vi "Sample_Data_Compute.vi"(8 "Data Array 2":dbl[][](array[numeric]), 11 "Data Array 1":dbl[][](array[numeric])) -> (0 "Cam2_Stats":cluster{"Mean_Area":i32, "Img_Count":u32} caption="Camera 2", 1 "Cam1_Stats":cluster{"Mean_Area":i32, "Img_Count":u32} caption="Camera 1", 3 "summaryData":T1)   [LabVIEW 2022 SP3]
uses:
  <vilib>/Analysis/NI_AALBase.lvlib
panel:
  in  "summaryData":T1
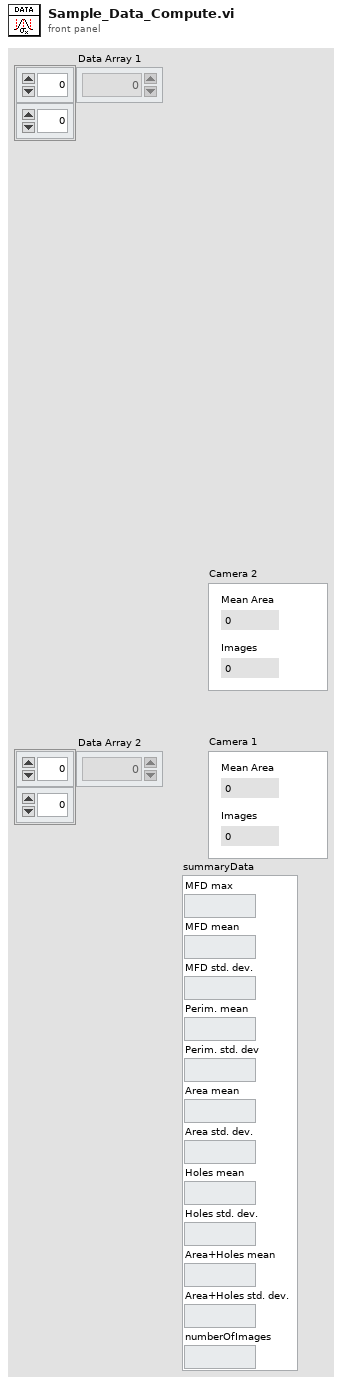
[diagram p1: front panel]
types:
  T1 = cluster{"MFD max":string, "MFD mean":string, "MFD std. dev.":string, "Perim. mean":string, "Perim. std. dev":string, "Area mean":string, "Area std. dev.":string, "Holes mean":string, "Holes std. dev.":string, "Area+Holes mean":string, "Area+Holes std. dev.":string, "numberOfImages":string}
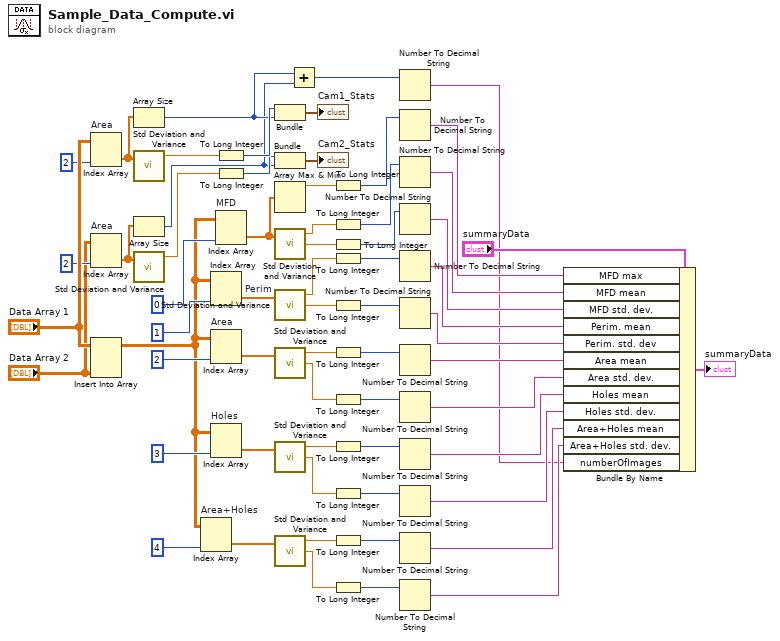
[diagram p0: block diagram]
diagram:
  n1 = Index Array "Area"(array="Data Array 1", index (col)=2 ("disabled index (col)")) -> (element=w11:dbl[])  [unwired: 1 in]
  n2 = Index Array "Area"(array="Data Array 2", index (col)=2 ("disabled index (col)")) -> (element=w10:dbl[])  [unwired: 1 in]
  n3 = Insert Into Array(array="Data Array 1", new element="Data Array 2") -> (w23:dbl[][])  [unwired: 2 in]
  n4 = Array Size(array=w11) -> (size(s)=w5:i32)
  n5 = call <vilib>:"Std Deviation and Variance.vi"("X"=w11) -> ("mean"=w17:dbl)  [unwired: 1 in, 2 out]
  n6 = Array Size(array=w10) -> (size(s)=w4:i32)
  n7 = call <vilib>:"Std Deviation and Variance.vi"("X"=w10) -> ("mean"=w13:dbl)  [unwired: 1 in, 2 out]
  n8 = Index Array "Area+Holes"(array=w23, index (col)=4 ("disabled index (col)")) -> (element=w18:dbl[])  [unwired: 1 in]
  n9 = Index Array "Perim"(array=w23, index (col)=1 ("disabled index (col)")) -> (element=w21:dbl[])  [unwired: 1 in]
  n10 = Index Array "Area"(array=w23, index (col)=2 ("disabled index (col)")) -> (element=w20:dbl[])  [unwired: 1 in]
  n11 = Index Array "Holes"(array=w23, index (col)=3 ("disabled index (col)")) -> (element=w19:dbl[])  [unwired: 1 in]
  n12 = To Long Integer(number=w17) -> (32bit integer=w9:i32)
  n13 = To Long Integer(number=w13) -> (32bit integer=w8:i32)
  n14 = Index Array "MFD"(array=w23, index (col)=0 ("disabled index (col)")) -> (element=w22:dbl[])  [unwired: 1 in]
  n15 = Bundle(w9, w5) -> (→"Cam1_Stats":cluster{i32, i32})  [unwired: 1 in]
  n16 = Bundle(w8, w4) -> (→"Cam2_Stats":cluster{i32, i32})  [unwired: 1 in]
  n17 = Array Max & Min(array=w22) -> (max value=w62:dbl)  [unwired: 3 out]
  n18 = call <vilib>:"Std Deviation and Variance.vi"("X"=w22) -> ("mean"=w33:dbl, "standard deviation"=w32:dbl)  [unwired: 1 in, 1 out]
  n19 = call <vilib>:"Std Deviation and Variance.vi"("X"=w21) -> ("mean"=w55:dbl, "standard deviation"=w52:dbl)  [unwired: 1 in, 1 out]
  n20 = call <vilib>:"Std Deviation and Variance.vi"("X"=w20) -> ("mean"=w50:dbl, "standard deviation"=w47:dbl)  [unwired: 1 in, 1 out]
  n21 = call <vilib>:"Std Deviation and Variance.vi"("X"=w19) -> ("mean"=w45:dbl, "standard deviation"=w41:dbl)  [unwired: 1 in, 1 out]
  n22 = call <vilib>:"Std Deviation and Variance.vi"("X"=w18) -> ("mean"=w38:dbl, "standard deviation"=w37:dbl)  [unwired: 1 in, 1 out]
  n23 = Add(x=w5, y=w4) -> (x+y=w3:i32)
  n24 = To Long Integer(number=w62) -> (32bit integer=w61:i32)
  n25 = To Long Integer(number=w33) -> (32bit integer=w35:i32)
  n26 = To Long Integer(number=w32) -> (32bit integer=w34:i32)
  n27 = To Long Integer(number=w55) -> (32bit integer=w60:i32)
  n28 = To Long Integer(number=w52) -> (32bit integer=w59:i32)
  n29 = To Long Integer(number=w50) -> (32bit integer=w58:i32)
  n30 = To Long Integer(number=w47) -> (32bit integer=w57:i32)
  n31 = To Long Integer(number=w45) -> (32bit integer=w56:i32)
  n32 = To Long Integer(number=w41) -> (32bit integer=w44:i32)
  n33 = To Long Integer(number=w38) -> (32bit integer=w43:i32)
  n34 = To Long Integer(number=w37) -> (32bit integer=w42:i32)
  n35 = Number To Decimal String(number=w3) -> (decimal integer string=w2:string)  [unwired: 1 in]
  n36 = Number To Decimal String(number=w61) -> (decimal integer string=w30:string)  [unwired: 1 in]
  n37 = Number To Decimal String(number=w35) -> (decimal integer string=w31:string)  [unwired: 1 in]
  n38 = Number To Decimal String(number=w34) -> (decimal integer string=w29:string)  [unwired: 1 in]
  n39 = Number To Decimal String(number=w60) -> (decimal integer string=w54:string)  [unwired: 1 in]
  n40 = Number To Decimal String(number=w59) -> (decimal integer string=w51:string)  [unwired: 1 in]
  n41 = Number To Decimal String(number=w58) -> (decimal integer string=w49:string)  [unwired: 1 in]
  n42 = Number To Decimal String(number=w57) -> (decimal integer string=w48:string)  [unwired: 1 in]
  n43 = Number To Decimal String(number=w56) -> (decimal integer string=w46:string)  [unwired: 1 in]
  n44 = Number To Decimal String(number=w44) -> (decimal integer string=w40:string)  [unwired: 1 in]
  n45 = Number To Decimal String(number=w43) -> (decimal integer string=w39:string)  [unwired: 1 in]
  n46 = Number To Decimal String(number=w42) -> (decimal integer string=w36:string)  [unwired: 1 in]
  n47 = Bundle By Name(cluster="summaryData", "MFD max"=w30, "MFD mean"=w31, "MFD std. dev."=w29, "Perim. mean"=w54, "Perim. std. dev"=w51, "Area mean"=w49, "Area std. dev."=w48, "Holes mean"=w46, "Holes std. dev."=w40, "Area+Holes mean"=w39, "Area+Holes std. dev."=w36, "numberOfImages"=w2) -> (→"summaryData":T1)
